vi "Siglent SDS 1000 2000 Series Edge Triggered Acquisition.vi"() -> ()   [LabVIEW 2021]
doc: "This example shows how to configure the oscilloscope to perform an edge-triggered waveform acquisition."
uses:
  <instrlib>/Siglent SDS 1000 2000 Series/Public/Configure/Configure Trigger (Edge).vi
  <instrlib>/Siglent SDS 1000 2000 Series/Public/Data/Read Waveform (Single).vi
  <instrlib>/Siglent SDS 1000 2000 Series/Siglent SDS 1000 2000 Series.lvlib
panel:
  in  "Vertical Coupling (0: A1M)":u16(ring) items=["A1M", "A50", "D1M", "D50", "Ground"]
  in  "Probe Attenuation (1X)":dbl=1.0
  in  "Vertical Range (1 V)":dbl=10.0
  in  "Trigger Level (0.0 V)":dbl
  in  "Timebase (0.0005 s)":dbl=0.0005
  out "Waveform Data":waveform(dbl)(graph)
  in  "Source (1: Channel 1)":u16(ring)=1 items=["Channel 1"=1, "Channel 2"=2, "Channel 3"=3, "Channel 4"=4]
  in  "VISA resource name":refnum<visa-resource-name>
  # "(c) 2015 SIGLENT TECHNOLOGIES CO., LTD.   ALL RIGHTS RESERVED."
  # "Note:\nThis VI will time out without acquiring any data if the input signal on  the selected channel does not cross 0 V trigger level with positive slope."
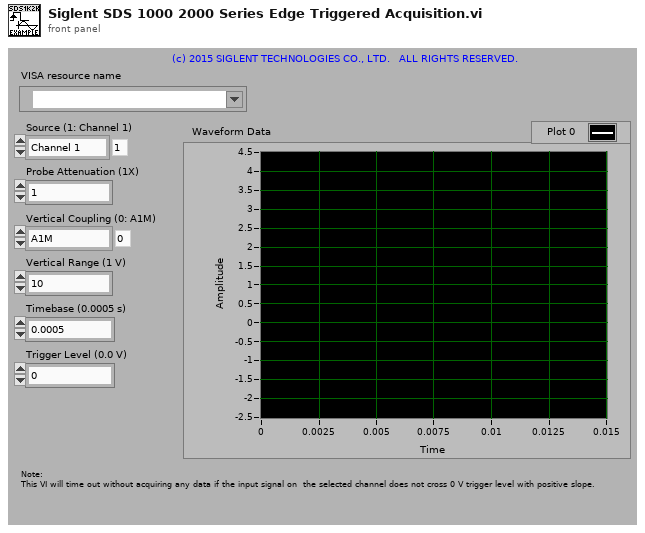
[diagram p1: front panel]
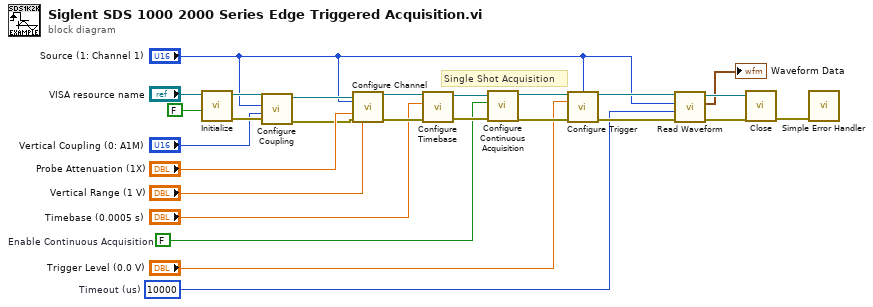
[diagram p0: block diagram]
diagram:
  w8 = u32 10000  # Timeout (us)
  w11 = FALSE  # Enable Continuous Acquisition
  # "Single Shot Acquisition"
  n1 = call <instrlib>:"Initialize.vi"("Reset (True)"=FALSE ("Reset? (T: Yes)"), "VISA resource name"="VISA resource name") -> ("error out"=w3:errorcluster, "VISA resource name out"=w6:refnum<visa-resource-name>)  [unwired: 8 in]
  n2 = call <instrlib>:"Configure Coupling.vi"("error in (no error)"=w3, "Vertical Coupling (0: A1M)"="Vertical Coupling (0: A1M)", "Channel (1: Channel 1)"="Source (1: Channel 1)", "VISA resource name"=w6) -> ("error out"=w4:errorcluster, "VISA resource name out"=w5:refnum<visa-resource-name>)  [unwired: 6 in]
  n3 = call <instrlib>:"Configure Channel.vi"("VISA resource name"=w5, "Channel (1: Channel 1)"="Source (1: Channel 1)", "Probe Attenuation (1X)"="Probe Attenuation (1X)", "error in (no error)"=w4, "Vertical Range (1.0 V)"="Vertical Range (1 V)") -> ("VISA resource name out"=w24:refnum<visa-resource-name>, "error out"=w25:errorcluster)  [unwired: 9 in]
  n4 = call <instrlib>:"Configure Timebase.vi"("error in (no error)"=w25, "Timebase (0.0005 s)"="Timebase (0.0005 s)", "VISA resource name"=w24) -> ("error out"=w13:errorcluster, "VISA resource name out"=w16:refnum<visa-resource-name>)  [unwired: 7 in]
  n5 = call <instrlib>:"Configure Continuous Acquisition.vi"("error in (no error)"=w13, "Enable Continuous Acquisition(T: On)"=w11, "VISA resource name"=w16) -> ("error out"=w14:errorcluster, "VISA resource name out"=w15:refnum<visa-resource-name>)  [unwired: 7 in]
  n6 = call-poly <instrlib>:"Configure Trigger.vi"("VISA resource name"=w15, "Trigger Source (1: Channel 1)"="Source (1: Channel 1)", "Trigger Level (0.0 V)"="Trigger Level (0.0 V)", "error in (no error)"=w14) -> ("VISA resource name out"=w18:refnum<visa-resource-name>, "error out"=w17:errorcluster)  [unwired: 10 in]
  n7 = call-poly <instrlib>:"Read Waveform.vi"("error in (no error)"=w17, "Timeout (10000 ms)"=w8, "Source (1: Channel 1)"="Source (1: Channel 1)", "VISA resource name"=w18) -> ("error out"=w20:errorcluster, "Waveform Data"=→"Waveform Data":waveform(dbl), "VISA resource name out"=w21:refnum<visa-resource-name>)  [unwired: 5 in]
  n8 = call <instrlib>:"Close.vi"("error in (no error)"=w20, "VISA resource name"=w21) -> ("error out"=w26:errorcluster)  [unwired: 9 in]
  n9 = call <vilib>:"Simple Error Handler.vi"("error in (no error)"=w26) -> ()  [unwired: 4 in, 5 out]
